vi "Edit.vi"() -> ()   [LabVIEW 2017]
panel:
  in  "Cancel":bool
  in  "valid":bool
  in  "Edit":bool
  in  "Delete Record":bool
  in  "Delete Image":bool
  in  "Previous 2":bool
  in  "Next 2":bool
  in  "Previous":bool
  in  "Next":bool
  out "Image":T1(plugin-control)
  in  "Data":string
  out "Location":string
  out "Name":string
  in  "Done":bool
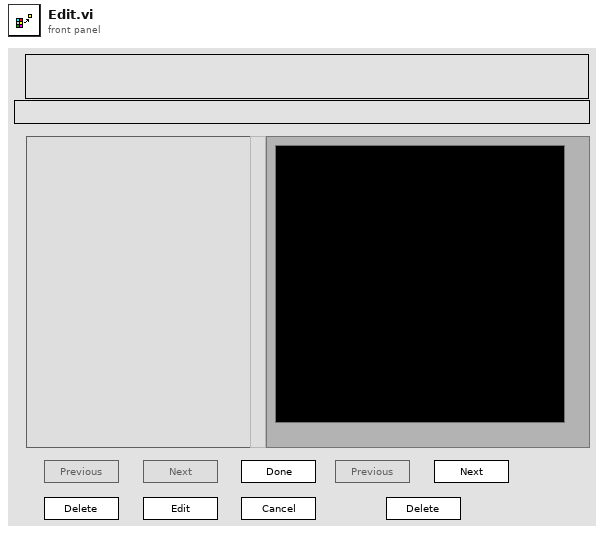
[diagram p1: front panel]
types:
  T1 = typedef "IMAQ Image.ctl" = refnum<image>
  T2 = enum8{"Enabled", "Disabled", "Disabled and Grayed Out"}
  T3 = typedef "Image Type" = u32
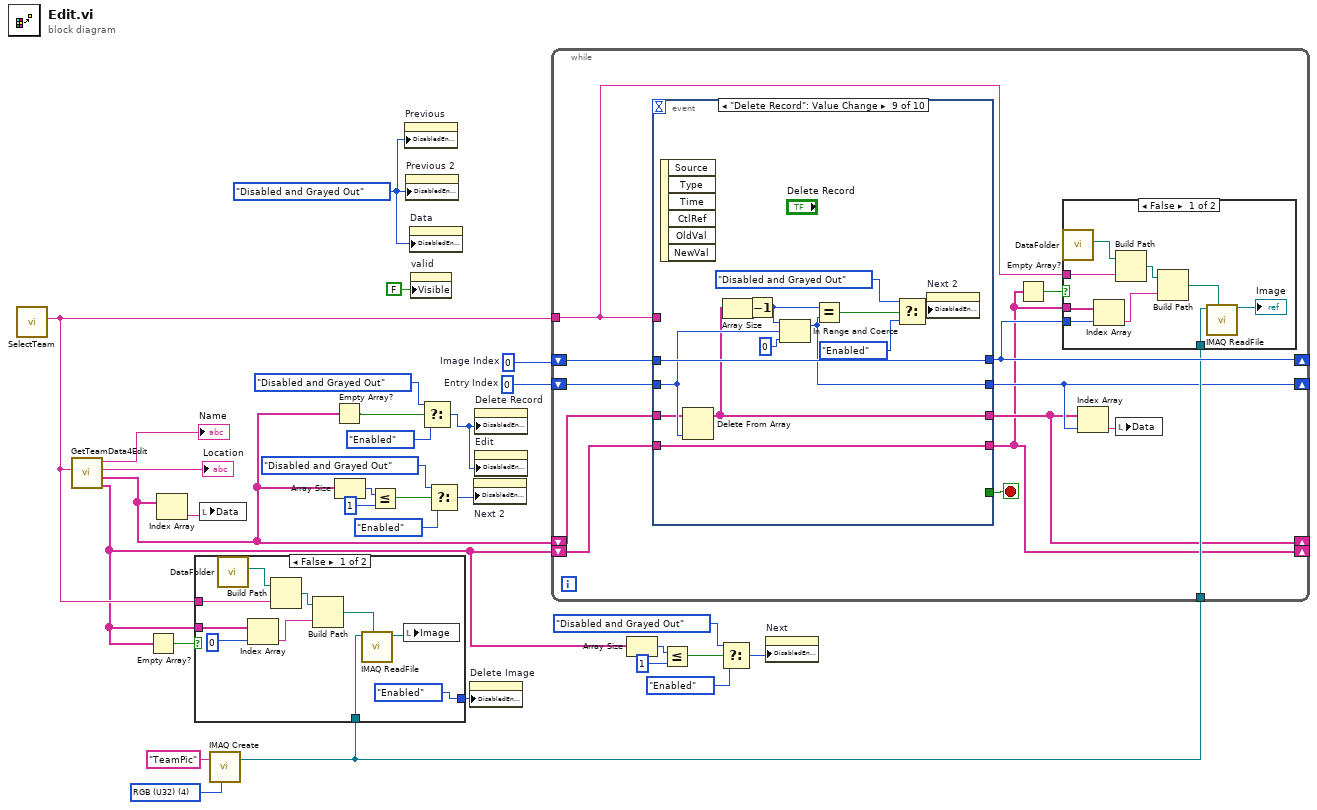
[diagram p0: block diagram]
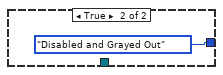
[diagram p2: hidden frame]
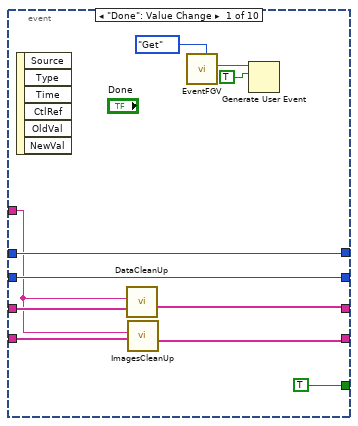
[diagram p4: hidden frame]
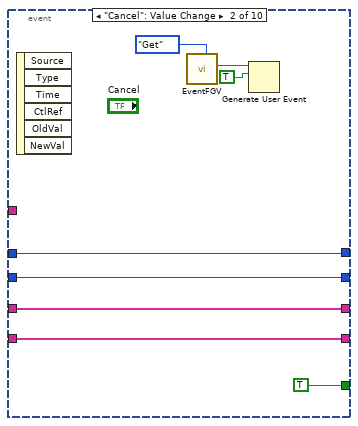
[diagram p5: hidden frame]
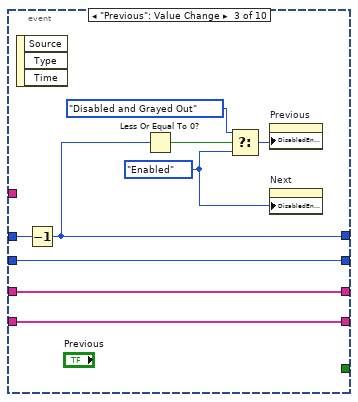
[diagram p6: hidden frame]
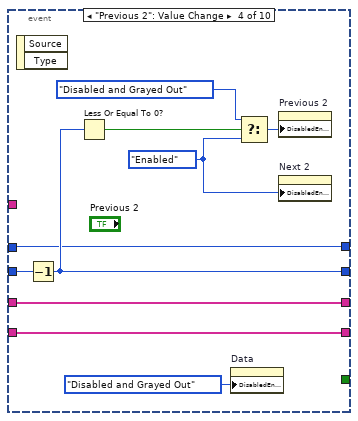
[diagram p7: hidden frame]
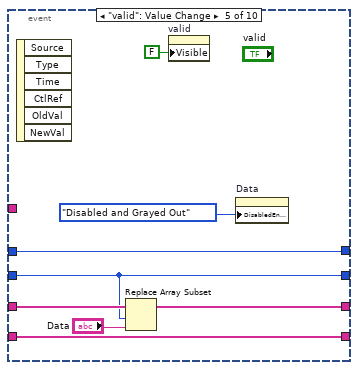
[diagram p8: hidden frame]
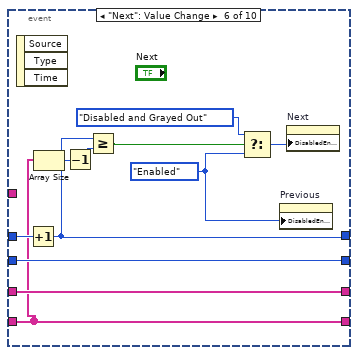
[diagram p9: hidden frame]
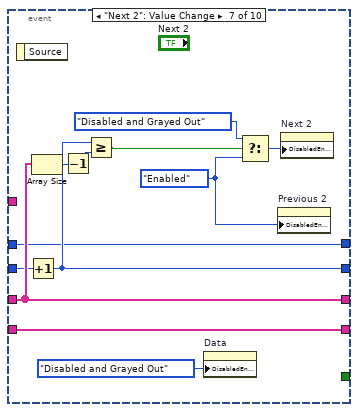
[diagram p10: hidden frame]
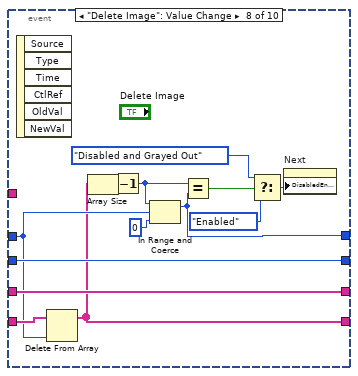
[diagram p11: hidden frame]
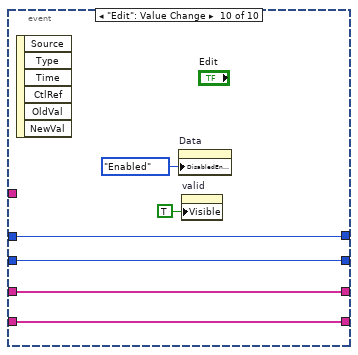
[diagram p12: hidden frame]
diagram:
  w11 = T2."Disabled and Grayed Out" ("Disabled")
  w18 = 0  # Entry Index
  w22 = T3 4 items=["Grayscale (U8)", "Grayscale (I16)", "Grayscale (SGL)", "Complex (CSG)", "RGB (U32)", "HSL (U32)", "RGB (U64)", "Grayscale (U16)"] ("Image Type")
  w31 = 0  # Image Index
  n1 = call "SelectTeam.vi"() -> ("Selected Team"=w21:string)  [unwired: 11 in]
  n2 = call "GetTeamData4Edit.vi"("Team #"=w21) -> ("Pictures"=w3:string[], "Data"=w4:string[], "Location"=→"Location":string, "Name"=→"Name":string)  [unwired: 7 in]
  n3 = Empty Array?(array=w3) -> (empty?=w20:bool)
  n4 = Index Array(array=w4) -> (element=w17:string)  [unwired: 1 in]
  n5 = local write "Data"(w17) -> ()
  n6 = call "IMAQ Create"("Image Name"="TeamPic", "Image Type"=w22) -> ("New Image"=w19:T1)  [unwired: 3 in, 1 out]
  n7 = case shown="False" w20 {
    tunnel: w3 -> [w37 _]
    tunnel: w21 -> [w35 _]
    tunnel: w19 -> [w33 _]
    tunnel: [T2."Enabled" ("Disabled") T2."Disabled and Grayed Out" ("Disabled")] -> w2
    frame False {
      n8 = call "DataFolder.vi"() -> ("appended path"=w38:path)  [unwired: 11 in]
      n9 = Index Array(array=w37, index=0) -> (element=w40:string)
      n10 = Build Path(base path=w38, name or relative path=w35) -> (appended path=w39:path)
      n11 = Build Path(base path=w39, name or relative path=w40) -> (appended path=w41:path)
      n12 = call "IMAQ ReadFile"("File Path"=w41, "Image"=w33) -> ("Image Out"=w34:T1)  [unwired: 5 in, 4 out]
      n13 = local write "Image"(w34) -> ()
    }
    frame True {
    }
  }
  n14 = Empty Array?(array=w4) -> (empty?=w5:bool)
  n15 = Array Size(array=w4) -> (size(s)=w28:i32)
  n16 = Less Or Equal?(x=w28, y=1) -> (x <= y?=w26:bool)
  n17 = property on="Previous" class="Bool"("DisabledEnum"=w11) -> ()  [unwired: 2 in, 2 out]
  n18 = property on="Previous 2" class="Bool"("DisabledEnum"=w11) -> ()  [unwired: 2 in, 2 out]
  n19 = property on="Data" class="Str"("DisabledEnum"=w11) -> ()  [unwired: 2 in, 2 out]
  n20 = property on="valid" class="Bool"("Visible"=FALSE) -> ()  [unwired: 2 in, 2 out]
  n21 = Select(t=T2."Disabled and Grayed Out" ("Disabled"), s=w5, f=T2."Enabled" ("Disabled")) -> (s? t:f=w6:T2)
  n22 = Select(t=T2."Disabled and Grayed Out" ("Disabled"), s=w26, f=T2."Enabled" ("Disabled")) -> (s? t:f=w9:T2)
  n23 = property on="Delete Image" class="Bool"("DisabledEnum"=w2) -> ()  [unwired: 2 in, 2 out]
  n24 = property on="Next 2" class="Bool"("DisabledEnum"=w9) -> ()  [unwired: 2 in, 2 out]
  n25 = property on="Delete Record" class="Bool"("DisabledEnum"=w6) -> ()  [unwired: 2 in, 2 out]
  n26 = property on="Edit" class="Bool"("DisabledEnum"=w6) -> ()  [unwired: 2 in, 2 out]
  n27 = while {
    tunnel: w21 -> [w52]
    shift-right: [w53] -> _
    shift-left: w31 -> [w54]
    tunnel: w19 -> [w51]
    shift-right: [w48] -> _
    shift-left: w18 -> [w49]
    shift-right: [w44] -> _
    shift-left: w4 -> [w47]
    shift-right: [w43] -> _
    shift-left: w3 -> [w45]
    stop <- w55 stop-if-true
    n28 = event shown="[8] \"Delete Record\": Value Change" {
      selector: _ -> [_ _ _ _ _ _ _ _ _ _]
      dyn-events: _ -> [_ _ _ _ _ _ _ _ _ _]
      timeout: _ -> [_ _ _ _ _ _ _ _ _ _]
      tunnel: [TRUE TRUE _ _ _ _ _ _ _ _] -> w55
      tunnel: w52 -> [w65 _ _ _ _ _ _ _ _ _]
      tunnel: [w71 w79 w91 w96 w110 w118 w125 w135 w156 w165] -> w53
      tunnel: w54 -> [w71 w79 w92 w96 w110 w121 w125 w140 w156 w165]
      tunnel: w47 -> [w67 w77 w85 w95 w109 w117 w132 w145 w151 w163]
      tunnel: [w70 w78 w86 w97 w106 w112 w126 w146 w148 w164] -> w48
      tunnel: w49 -> [w70 w78 w86 w98 w106 w112 w127 w146 w152 w164]
      tunnel: [w66 w77 w85 w95 w107 w117 w132 w145 w150 w163] -> w44
      tunnel: [w68 w76 w84 w94 w108 w111 w123 w138 w149 w162] -> w43
      tunnel: w45 -> [w69 w76 w84 w94 w108 w111 w123 w144 w149 w162]
      event "Done": Value Change {
        n29 = event-data() -> ()  [unwired: 1 in, 6 out]
        n30 = call "DataCleanUp.vi"("Data in"=w67, "Team"=w65) -> ("Data out"=w66:string[])  [unwired: 9 in]
        n31 = call "ImagesCleanUp.vi"("Pictures in"=w69, "Team"=w65) -> ("Pictures out"=w68:string[])  [unwired: 9 in]
        n32 = call "EventFGV.vi"("Action"=enum16{"Set", "Get"}."Get") -> ("user event out"=w75:refnum<user-event>)  [unwired: 10 in]
        n33 = Generate User Event(user event=w75, event data cluster=TRUE ("event data")) -> ()  [unwired: 2 in, 2 out]
      }
      event "Cancel": Value Change {
        n34 = event-data() -> ()  [unwired: 1 in, 6 out]
        n35 = call "EventFGV.vi"("Action"=enum16{"Set", "Get"}."Get") -> ("user event out"=w83:refnum<user-event>)  [unwired: 10 in]
        n36 = Generate User Event(user event=w83, event data cluster=TRUE ("event data")) -> ()  [unwired: 2 in, 2 out]
      }
      event "Previous": Value Change {
        w87 = T2."Enabled" ("Disabled")
        n37 = event-data() -> ()  [unwired: 1 in, 3 out]
        n38 = Decrement(x=w92) -> (x-1=w91:i32)
        n39 = Less Or Equal To 0?(x=w91) -> (x <= 0?=w88:bool)
        n40 = Select(t=T2."Disabled and Grayed Out" ("Disabled"), s=w88, f=w87) -> (s? t:f=w89:T2)
        n41 = property on="Previous" class="Bool"("DisabledEnum"=w89) -> ()  [unwired: 2 in, 2 out]
        n42 = property on="Next" class="Bool"("DisabledEnum"=w87) -> ()  [unwired: 2 in, 2 out]
      }
      event "Previous 2": Value Change {
        w100 = T2."Enabled" ("Disabled")
        n43 = event-data() -> ()  [unwired: 1 in, 2 out]
        n44 = Decrement(x=w98) -> (x-1=w97:i32)
        n45 = Less Or Equal To 0?(x=w97) -> (x <= 0?=w101:bool)
        n46 = property on="Data" class="Str"("DisabledEnum"=T2."Disabled and Grayed Out" ("Disabled")) -> ()  [unwired: 2 in, 2 out]
        n47 = Select(t=T2."Disabled and Grayed Out" ("Disabled"), s=w101, f=w100) -> (s? t:f=w99:T2)
        n48 = property on="Previous 2" class="Bool"("DisabledEnum"=w99) -> ()  [unwired: 2 in, 2 out]
        n49 = property on="Next 2" class="Bool"("DisabledEnum"=w100) -> ()  [unwired: 2 in, 2 out]
      }
      event "valid": Value Change {
        n50 = event-data() -> ()  [unwired: 1 in, 6 out]
        n51 = Replace Array Subset(array=w109, new element="Data", index=w106) -> (w107:string[])
        n52 = property on="valid" class="Bool"("Visible"=FALSE) -> ()  [unwired: 2 in, 2 out]
        n53 = property on="Data" class="Str"("DisabledEnum"=T2."Disabled and Grayed Out" ("Disabled")) -> ()  [unwired: 2 in, 2 out]
      }
      event "Next": Value Change {
        w113 = T2."Enabled" ("Disabled")
        n54 = event-data() -> ()  [unwired: 1 in, 3 out]
        n55 = Increment(x=w121) -> (x+1=w118:i32)
        n56 = Array Size(array=w111) -> (size(s)=w116:i32)
        n57 = Decrement(x=w116) -> (x-1=w114:i32)
        n58 = Greater Or Equal?(x=w118, y=w114) -> (x >= y?=w115:bool)
        n59 = Select(t=T2."Disabled and Grayed Out" ("Disabled"), s=w115, f=w113) -> (s? t:f=w119:T2)
        n60 = property on="Previous" class="Bool"("DisabledEnum"=w113) -> ()  [unwired: 2 in, 2 out]
        n61 = property on="Next" class="Bool"("DisabledEnum"=w119) -> ()  [unwired: 2 in, 2 out]
      }
      event "Next 2": Value Change {
        w128 = T2."Enabled" ("Disabled")
        n62 = event-data() -> ()  [unwired: 1 in, 1 out]
        n63 = Increment(x=w127) -> (x+1=w126:i32)
        n64 = Array Size(array=w132) -> (size(s)=w131:i32)
        n65 = Decrement(x=w131) -> (x-1=w129:i32)
        n66 = Greater Or Equal?(x=w126, y=w129) -> (x >= y?=w130:bool)
        n67 = property on="Data" class="Str"("DisabledEnum"=T2."Disabled and Grayed Out" ("Disabled")) -> ()  [unwired: 2 in, 2 out]
        n68 = Select(t=T2."Disabled and Grayed Out" ("Disabled"), s=w130, f=w128) -> (s? t:f=w124:T2)
        n69 = property on="Previous 2" class="Bool"("DisabledEnum"=w128) -> ()  [unwired: 2 in, 2 out]
        n70 = property on="Next 2" class="Bool"("DisabledEnum"=w124) -> ()  [unwired: 2 in, 2 out]
      }
      event "Delete Image": Value Change {
        n71 = event-data() -> ()  [unwired: 1 in, 6 out]
        n72 = Delete From Array(array=w144, index=w140) -> (array with subset deleted=w138:string[])  [unwired: 1 in, 1 out]
        n73 = Array Size(array=w138) -> (size(s)=w137:i32)
        n74 = Decrement(x=w137) -> (x-1=w134:i32)
        n75 = In Range and Coerce(upper limit=w134, x=w140, lower limit=0) -> (coerced(x)=w135:i32)  [unwired: 1 out]
        n76 = Equal?(x=w134, y=w135) -> (x = y?=w136:bool)
        n77 = Select(t=T2."Disabled and Grayed Out" ("Disabled"), s=w136, f=T2."Enabled" ("Disabled")) -> (s? t:f=w143:T2)
        n78 = property on="Next" class="Bool"("DisabledEnum"=w143) -> ()  [unwired: 2 in, 2 out]
      }
      event "Delete Record": Value Change {
        n79 = event-data() -> ()  [unwired: 1 in, 6 out]
        n80 = Delete From Array(array=w151, index=w152) -> (array with subset deleted=w150:string[])  [unwired: 1 in, 1 out]
        n81 = Array Size(array=w150) -> (size(s)=w154:i32)
        n82 = Decrement(x=w154) -> (x-1=w147:i32)
        n83 = In Range and Coerce(upper limit=w147, x=w152, lower limit=0) -> (coerced(x)=w148:i32)  [unwired: 1 out]
        n84 = Equal?(x=w147, y=w148) -> (x = y?=w153:bool)
        n85 = Select(t=T2."Disabled and Grayed Out" ("Disabled"), s=w153, f=T2."Enabled" ("Disabled")) -> (s? t:f=w159:T2)
        n86 = property on="Next 2" class="Bool"("DisabledEnum"=w159) -> ()  [unwired: 2 in, 2 out]
      }
      event "Edit": Value Change {
        n87 = event-data() -> ()  [unwired: 1 in, 6 out]
        n88 = property on="Data" class="Str"("DisabledEnum"=T2."Enabled" ("Disabled")) -> ()  [unwired: 2 in, 2 out]
        n89 = property on="valid" class="Bool"("Visible"=TRUE) -> ()  [unwired: 2 in, 2 out]
      }
    }
    n90 = Empty Array?(array=w43) -> (empty?=w50:bool)
    n91 = case shown="False" w50 {
      tunnel: w53 -> [w64 _]
      tunnel: w43 -> [w63 _]
      tunnel: w52 -> [w61 _]
      tunnel: w51 -> [w56 _]
      frame False {
        n92 = call "DataFolder.vi"() -> ("appended path"=w62:path)  [unwired: 11 in]
        n93 = Index Array(array=w63, index=w64) -> (element=w59:string)
        n94 = Build Path(base path=w62, name or relative path=w61) -> (appended path=w60:path)
        n95 = Build Path(base path=w60, name or relative path=w59) -> (appended path=w57:path)
        n96 = call "IMAQ ReadFile"("File Path"=w57, "Image"=w56) -> ("Image Out"=→"Image":T1)  [unwired: 5 in, 4 out]
      }
      frame True {
      }
    }
    n97 = Index Array(array=w44, index=w48) -> (element=w46:string)
    n98 = local write "Data"(w46) -> ()
  }
  n99 = Array Size(array=w3) -> (size(s)=w12:i32)
  n100 = Less Or Equal?(x=w12, y=1) -> (x <= y?=w14:bool)
  n101 = Select(t=T2."Disabled and Grayed Out" ("Disabled"), s=w14, f=T2."Enabled" ("Disabled")) -> (s? t:f=w10:T2)
  n102 = property on="Next" class="Bool"("DisabledEnum"=w10) -> ()  [unwired: 2 in, 2 out]
